vi "Timer.vi"(7 "Waveform Chart":refnum<vi>, 8 "error in (no error)":errorcluster, 9 "window":dbl[unit], 10 "dt":dbl[unit], 11 "Timer in":refnum<class "Timer.lvclass">) -> (0 "error out":errorcluster, 3 "Timer out":refnum<class "Timer.lvclass">)   [LabVIEW 2023, in "Timer.lvclass"]
uses:
  Timer.lvclass
  Timer.lvclass/Timer.ctl
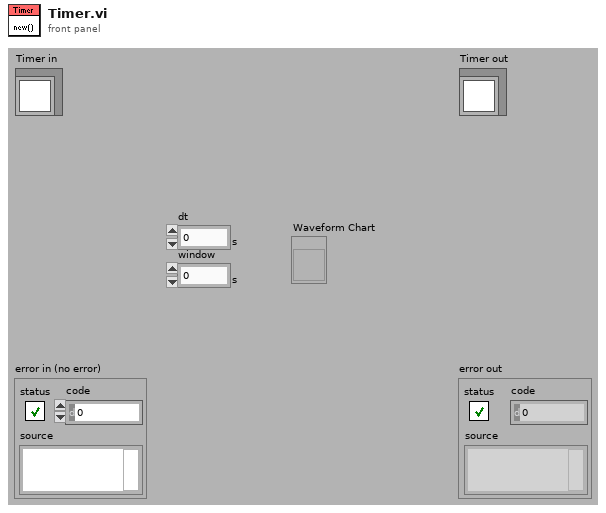
[diagram p1: front panel]
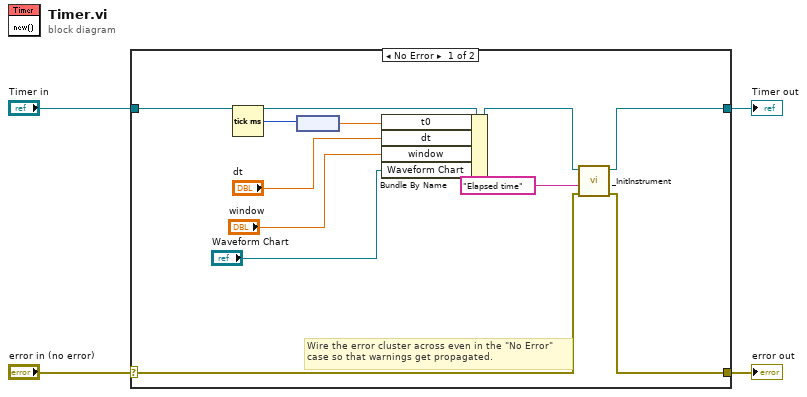
[diagram p0: block diagram]
diagram:
  n1 = case shown="No Error" "error in (no error)" {
    selector: "error in (no error)" -> [w9 w17]
    tunnel: [w6 w17] -> w3
    tunnel: [w7 w16] -> w1
    tunnel: "Timer in" -> [w15 w16]
    frame No Error {
      # "Wire the error cluster across even in the \"No Error\"\ncase so that warnings get propagated."
      n2 = Tick Count (ms)() -> (millisecond timer value=w12:u32)
      n3 = node(w12) -> (w13:dbl[unit])
      n4 = Bundle By Name(cluster=w15, "t0"=w13, "dt"="dt", "window"="window", "Waveform Chart"="Waveform Chart") -> (w8:refnum<class "Timer.lvclass">)
      n5 = call-dynamic "_InitInstrument.vi"("error in (no error)"=w9, "Name"="Elapsed time", "Instrument in"=w8) -> ("error out"=w6:errorcluster, "Instrument out"=w7:refnum<class "Timer.lvclass">)  [unwired: 3 in, 4 out]
    }
    frame Error {
    }
  }
  "error out" <- w3
  "Timer out" <- w1
